vi "Mask Write Holding Register.vi"(4 "OR Mask":u16, 6 "AND Mask":u16, 8 "error in":errorcluster, 10 "address":u16, 11 "Modbus instance in":refnum<class "Modbus Master.lvclass">) -> (0 "error out":errorcluster, 3 "Modbus instance out":refnum<class "Modbus Master.lvclass">)   [LabVIEW 2014, in "MyLib.lvlib" / "Modbus Master.lvclass"]
doc: "Writes the masked value of a single register using an <b>AND mask</b> and an <b>OR mask</b> using the equation below:\nResult=(Current Value AND AndMask) OR (OrMask AND !AndMask)"
uses:
  Modbus Master.lvclass
  Modbus Master.lvclass/Modbus Master.ctl
  Modbus API.lvclass/Modbus API.ctl
  Transmission Data Unit/Transmission Data Unit.lvclass
  Master Function Definition/Master Function Definition.lvclass
  Modbus API.lvclass
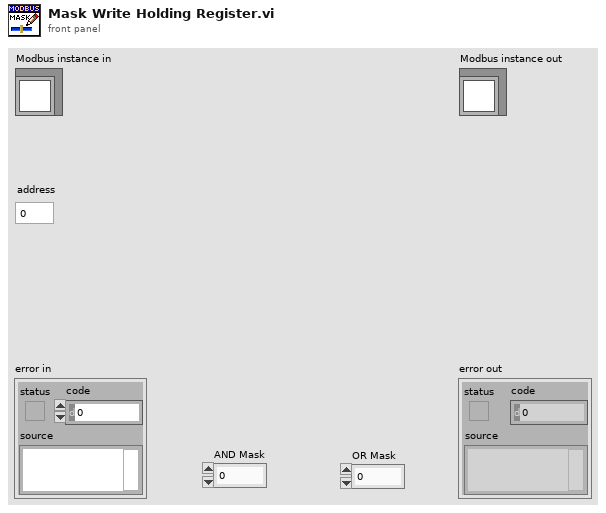
[diagram p1: front panel]
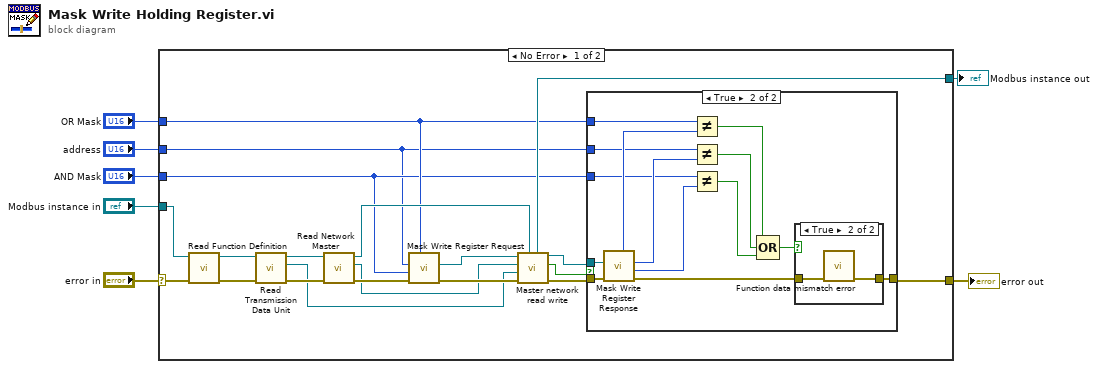
[diagram p0: block diagram]
diagram:
  n1 = case shown="No Error" "error in" {
    selector: "error in" -> [w17 w46]
    tunnel: "Modbus instance in" -> [w15 w47]
    tunnel: [w22 w47] -> w6
    tunnel: [w26 w46] -> w5
    tunnel: "OR Mask" -> [w11 _]
    tunnel: "address" -> [w9 _]
    tunnel: "AND Mask" -> [w10 _]
    frame No Error {
      n2 = call "Read Function Definition.vi"("error in"=w17, "Modbus master in"=w15) -> ("error out"=w20:errorcluster, "Modbus master out"=w19:refnum<class "Modbus Master.lvclass">)  [unwired: 7 in, 1 out]
      n3 = call "Read Transmission Data Unit.vi"("error in"=w20, "Modbus instance in"=w19) -> ("error out"=w18:errorcluster, "transmission data unit"=w13:refnum<class "Transmission Data Unit.lvclass">, "Modbus instance out"=w21:refnum<class "Modbus Master.lvclass">)  [unwired: 7 in]
      n4 = call "Read Network Master.vi"("error in"=w18, "Modbus master in"=w21) -> ("error out"=w16:errorcluster, "network master"=w12:refnum<class "Network Master.lvclass">, "Modbus master out"=w14:refnum<class "Modbus Master.lvclass">)  [unwired: 7 in]
      n5 = call "Mask Write Register Request.vi"("OR mask"=w11, "error in"=w16, "AND mask"=w10, "Starting Address"=w9) -> ("error out"=w27:errorcluster, "modbus data unit out"=w24:refnum<class "Modbus Data Unit.lvclass">)  [unwired: 6 in]
      n6 = call "Master network read write.vi"("Modbus master in"=w14, "error in"=w27, "transmission data unit in"=w13, "network master in"=w12, "Modbus data unit in"=w24) -> ("error out"=w25:errorcluster, "PDU Valid?"=w8:bool, "Modbus data unit out"=w23:refnum<class "Modbus Data Unit.lvclass">, "Modbus master out"=w22:refnum<class "Modbus Master.lvclass">)  [unwired: 3 in]
      n7 = case shown="True" w8 {
        tunnel: [w28 w40] -> w26
        tunnel: w25 -> [w28 w37]
        tunnel: w23 -> [_ w36]
        tunnel: w11 -> [_ w31]
        tunnel: w10 -> [_ w30]
        tunnel: w9 -> [_ w29]
        frame False {
        }
        frame True {
          n8 = call "Mask Write Register Response.vi"("error in"=w37, "modbus data unit in"=w36) -> ("error out"=w35:errorcluster, "AND mask"=w38:u16, "Address"=w39:u16, "OR mask"=w32:u16)  [unwired: 6 in]
          n9 = Not Equal?(x=w31, y=w32) -> (x != y?=w33:bool)
          n10 = Not Equal?(x=w29, y=w39) -> (x != y?=w34:bool)
          n11 = Not Equal?(x=w30, y=w38) -> (x != y?=w42:bool)
          n12 = Compound Arithmetic op=OR(w33, w34, w42) -> (w41:bool)
          n13 = case shown="True" w41 {
            tunnel: [w43 w45] -> w40
            tunnel: w35 -> [w43 w44]
            frame False {
            }
            frame True {
              n14 = call "Function data mismatch error.vi"("error in (no error)"=w44) -> ("error out"=w45:errorcluster)  [unwired: 10 in]
            }
          }
        }
      }
    }
    frame Error {
    }
  }
  "error out" <- w5
  "Modbus instance out" <- w6
